vi "General Cosine Window (CDB).vi"(2 "Cosine Coefficients":dbl[](array[numeric]), 3 "X":cdb[](array[numeric])) -> (0 "error":i32, 1 "Windowed X":cdb[](array[numeric]))   [LabVIEW 2018, in "NI_AALPro.lvlib"]
doc: "Applies a general cosine window to the input signal <B>X</B>. Wire data to the <B>X</B> input to determine the polymorphic instance to use or manually select the instance."
uses:
  <vilib>/Analysis/NI_AALPro.lvlib
  <resource>/lvanlys.dll
panel:
  # "General Cosine Window"
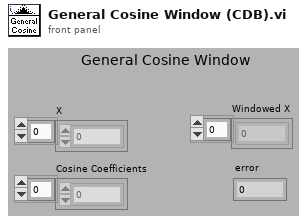
[diagram p1: front panel]
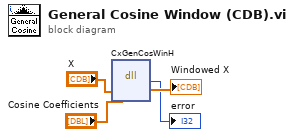
[diagram p0: block diagram]
diagram:
  n1 = dll-call lib="C:/Program Files (x86)/National Instruments/LabVIEW 2018/resource/lvanlys.*" fn="CxGenCosWinH"("X"="X", "Cosine Coefficients"="Cosine Coefficients") -> (→"error":i32, "X"=→"Windowed X":cdb[])  [unwired: 4 in, 2 out]
